vi "IR+Arduino+LabView.vi"() -> ()   [LabVIEW 2019]
uses:
  <vilib>/MakerHub/LINX/Public/Peripherals/Digital/Digital Read 1 Chan.vi
  <vilib>/MakerHub/LINX/Public/Peripherals/Digital/Digital Read N Chans.vi
  <vilib>/MakerHub/LINX/Private/Local IO/LinxDigitalRead.vi
  <vilib>/MakerHub/LINX/Public/Utilities/Check Channel.vi
  <vilib>/Utility/file.llb/Write Delimited Spreadsheet (string).vi
  <vilib>/MakerHub/LINX/Public/Utilities/Open Serial.vi
  <vilib>/MakerHub/LINX/Private/Utilties/Generate Error.vi
  <vilib>/Utility/file.llb/Write Delimited Spreadsheet (I64).vi
  <vilib>/MakerHub/LINX/LMH-LINX.lvlib
panel:
  in  "?":bool
  in  "file path (For sensor data)":path=path "C:/Users/aslam/Desktop/Sensor data.xls"
  out "?":i16
  out "Sensor Status":dbl
  out "IR Sensor status":bool
  in  "DI Channel":u8=8
  in  "Serial Port":refnum<visa-resource-name>="COM3"
  # "Feedind the IR sensor data to Excel file using Arduino UNO R3"
  # "Control panel"
  # "Output Data"
  # "Number of people pass through the Gate"
  # "Arduino configurations"
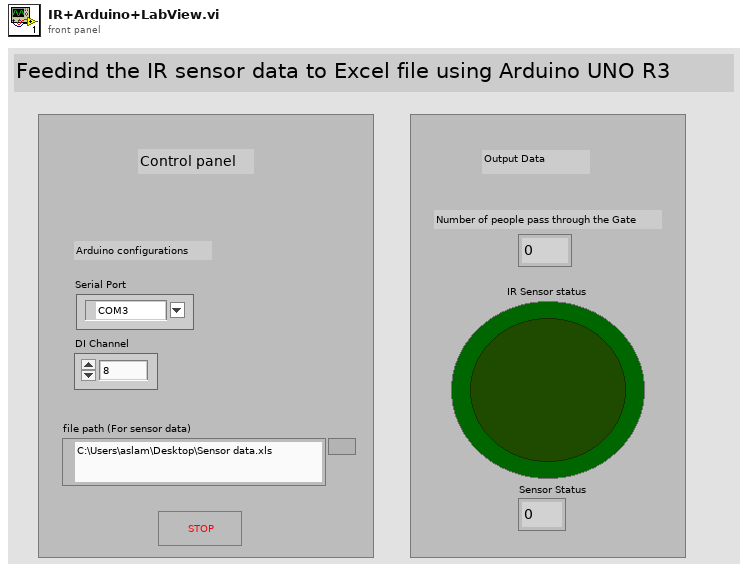
[diagram p1: front panel]
types:
  T1 = typedef "LMH-LINX.lvlib/LINX Ref.ctl" = cluster{"IO":T2, "Interface":T3, "LINX Device Config":T4}
  T2 = typedef "LMH-LINX.lvlib/Platform.ctl" = enum16{"Remote", "Local"}
  T3 = typedef "LMH-LINX.lvlib/Interface.ctl" = enum16{"Serial", "TCP"}
  T4 = typedef "LMH-LINX.lvlib/Device.lvlib/LINX Device Config.ctl" = cluster{"Interface":T3, "COM Port":refnum<visa-resource-name>, "TCP Configuration":T5, "Device Family":u8, "Device ID":u8, "Device Name":string, "TCP Ref":refnum<k5>, "Channels":T6}
  T5 = typedef "LMH-LINX.lvlib/Device.lvlib/TCP Config.ctl" = cluster{"IP Address":string, "Port":u16}
  T6 = typedef "LMH-LINX.lvlib/Channels.ctl" = cluster{"DI":u8[], "DO":u8[], "AI":u8[], "AO":u8[], "PWM":u8[], "QE":u8[], "UART":u8[], "I2C 2":u8[], "SPI":u8[], "CAN":u8[], "Servo":u8[], "AI Ref (V)":dbl, "AI Resolution (Bits)":u8, "AO Ref (V)":dbl, "AO Resolution (Bits)":u8}
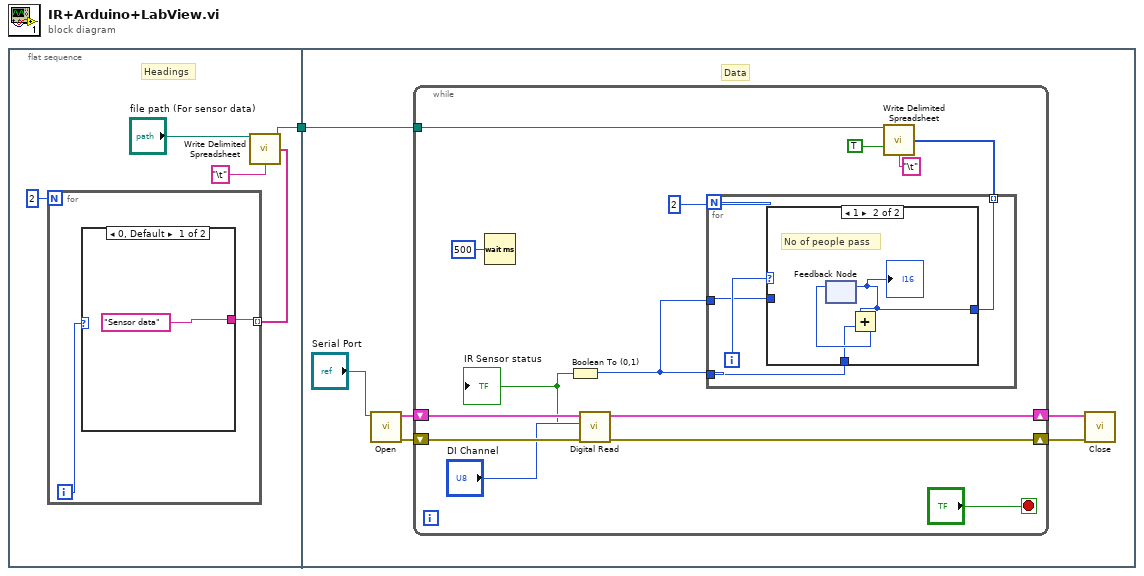
[diagram p0: block diagram]
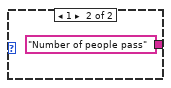
[diagram p2: hidden frame]
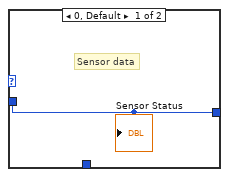
[diagram p3: hidden frame]
diagram:
  n1 = flat-sequence {
    tunnel: [w2] -> w1
    tunnel: w1 -> [w12]
    frame #0 {
      # "Headings"
      n2 = for {
        N: 2 -> [_]
        tunnel: [w7] -> w5 mode=indexing
        i -> [w8]
        n3 = case shown="0, Default" w8 {
          tunnel: ["Sensor data" "Number of people pass"] -> w7
          frame 0, Default {
          }
          frame 1 {
          }
        }
      }
      n4 = call-poly <vilib>:"Write Delimited Spreadsheet.vi"("file path (dialog if empty)"="file path (For sensor data)", "1D data"=w5, "delimiter (\\t)"="\t" ("delimiter (\\t)")) -> ("new file path (Not A Path if cancelled)"=w2:path)  [unwired: 11 in, 1 out]
    }
    frame #1 {
      # "Data"
      n5 = call-poly <vilib>:"Open.vi"("Serial Port"="Serial Port") -> ("Error Out"=w14:errorcluster, "LINX Resource"=w13:T1)  [unwired: 8 in, 1 out]
      n6 = while {
        shift-right: [w30] -> w16
        shift-left: w14 -> [w28]
        shift-right: [w29] -> w15
        shift-left: w13 -> [w27]
        tunnel: w12 -> [w22]
        stop <- "?" stop-if-true
        n7 = Wait (ms)(milliseconds to wait=u32 500) -> ()  [unwired: 1 out]
        n8 = call-poly <vilib>:"Digital Read.vi"("Error In"=w28, "DI Channel"="DI Channel", "LINX Resource"=w27) -> ("Error Out"=w30:errorcluster, "DI Value"=w25:bool, "LINX Resource"=w29:T1)  [unwired: 6 in]
        "IR Sensor status" <- w25
        n9 = Boolean To (0,1)(Boolean=w25) -> (0, 1=w20:i16)
        n10 = for {
          N: 2 -> [_]
          tunnel: w20 -> [w33]
          tunnel: w20 -> [w32]
          tunnel: [w31] -> w19 mode=indexing
          i -> [w34]
          n11 = case shown="1" w34 {
            tunnel: w33 -> [w35 _]
            tunnel: w32 -> [_ w36]
            tunnel: [w35 w37] -> w31
            frame 0, Default {
              # "Sensor data"
              "Sensor Status" <- w35
            }
            frame 1 {
              # "No of people pass"
              n12 = feedback #1() -> (w37:i16)  [unwired: 1 in]
              "?" <- w37
              n13 = Add(x=w37, y=w36) -> (x+y=w38:i16)
              n14 = feedback-in #1(w38) -> ()
            }
          }
        }
        n15 = call-poly <vilib>:"Write Delimited Spreadsheet.vi"("file path (dialog if empty)"=w22, "1D data"=w19, "append to file? (new file:F)"=TRUE, "delimiter (\\t)"="\t" ("delimiter (\\t)")) -> ()  [unwired: 10 in, 2 out]
      }
      n16 = call <vilib>:"Close.vi"("Error In"=w16, "LINX Resource"=w15) -> ()  [unwired: 9 in, 1 out]
    }
  }
